vi "hold eol seesion decision.vi"(9 "Communication Type":T2, 10 "Sequence State in":T3, 11 "Motion Status.Motion":T1) -> (2 "Sequence State out":T3, 3 "Event queue out":string[](array[string]))   [LabVIEW 2018]
uses:
  02.Type Def's/sequence state.ctl
  05.UserVI's/sequence/type defs/Sequence Info.ctl
  02.Type Def's/All Communication Types.ctl
  02.Type Def's/All Motions.ctl
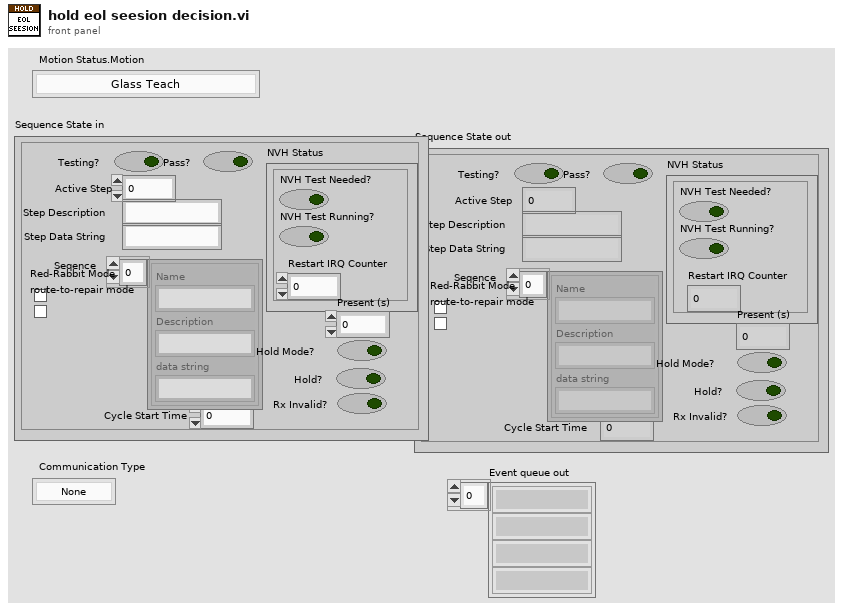
[diagram p1: front panel]
types:
  T1 = typedef "All Motions.ctl" = enum16{"Glass Teach", "Glass Slide Open", "Glass Slide Close", "Glass Vent Open", "Glass Vent Close", "Sunshade Teach", "Sunshade Open", "Sunshade Close", "Idle", "Sunshade Open 2", "Sunshade Close 2", "Glass Slide Open Sunshade Open", "Glass Slide Open Sunshade Close", "Glass Slide Close Sunshade Open", "Glass Slide Close Sunshade Close", "Glass Vent Open Sunshade Open", "Glass Vent Open Sunshade Close", "Glass Vent Close Sunshade Open", "Glass Vent Close Sunshade Close", "Express Glass Slide Open", "Express Glass Slide Close", "Express Glass Vent Open", "Express Glass Vent Close", "Express Sunshade Open", "Express Sunshade Close", "Express Sunshade Open 2", "Express Sunshade Close 2", "Express Glass Slide Open Sunshade Open", "Express Glass Slide Open Sunshade Close", "Express Glass Slide Close Sunshade Open", "Express Glass Slide Close Sunshade Close", "Express Glass Vent Open Sunshade Open", "Express Glass Vent Open Sunshade Close", "Express Glass Vent Close Sunshade Open", "Express Glass Vent Close Sunshade Close", "Goto Position Glass", "Goto Position Sunshade", "Sunshade Teach 2"}
  T2 = typedef "All Communication Types.ctl" = enum16{"None", "CAN", "RS 232", "RS 232 LIN", "GM LIN", "SnT LIN", "K Line", "Robel CAN", "P42M-Continental", "Inalfa SCU LIN", "Spare 3"}
  T3 = typedef "sequence state.ctl" = cluster{"Step Description":string, "Cycle Start Time":u32, "Step Data String":string, "Pass?":bool, "Seqence":T4[], "Active Step":u8, "Testing?":bool, "Red-Rabbit Mode":bool, "route-to-repair mode":bool, "NVH Status":cluster{"Restart IRQ Counter":u8, "NVH Test Needed?":bool, "NVH Test Running?":bool}, "Present (s)":dbl, "Hold Mode?":bool, "Hold?":bool, "Rx Invalid?":bool}
  T4 = typedef "Sequence Info.ctl" = cluster{"Name":string, "Description":string, "data string":string}
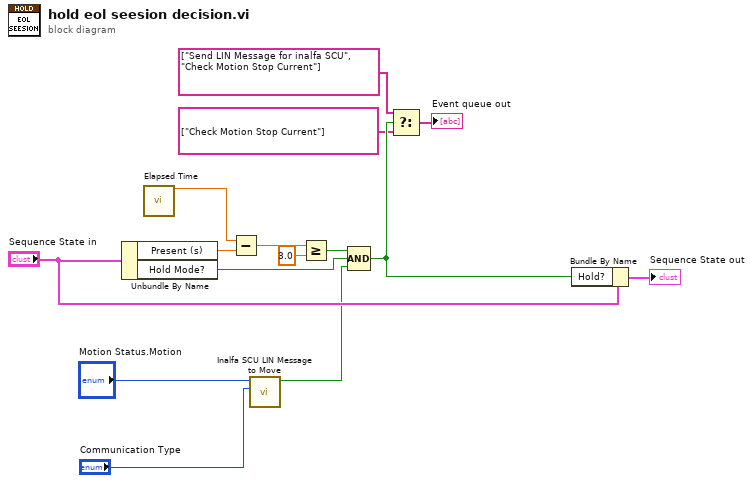
[diagram p0: block diagram]
diagram:
  n1 = Unbundle By Name("Sequence State in") -> ("Present (s)"=w4:dbl, "Hold Mode?"=w9:bool)
  n2 = call "Elapsed Time"() -> ("Present (s)"=w5:dbl)  [unwired: 12 in, 7 out]
  n3 = Subtract(x=w5, y=w4) -> (x-y=w12:dbl)
  n4 = call "Inalfa SCU LIN Message to Move.vi"("Communication Type"="Communication Type", "Motion"="Motion Status.Motion") -> ("Have Swtich?"=w1:bool)  [unwired: 9 in]
  n5 = Greater Or Equal?(x=w12, y=3.0) -> (x >= y?=w10:bool)
  n6 = Compound Arithmetic op=AND(w10, w9, w1) -> (w8:bool)
  n7 = Select(t=string[] ["Send LIN Message for inalfa SCU", "Check Motion Stop Current"] ("Events to Insert"), s=w8, f=string[] ["Check Motion Stop Current"] ("Events to Insert")) -> (s? t:f=→"Event queue out":string[])
  n8 = Bundle By Name(cluster="Sequence State in", "Hold?"=w8) -> (→"Sequence State out":T3)
